vi "Integration Time.vi"(8 "error in (no error)":errorcluster, 10 "Integration Time (0:Short)":u32(ring) items=["Short", "Medium", "Long"], 11 "VISA resource name":refnum<visa-resource-name>) -> (0 "error out":errorcluster, 3 "VISA resource name out":refnum<visa-resource-name>)   [LabVIEW 2017, in "Agilent 4194.lvlib"]
doc: "This function specifies the specifies the integration time."
uses:
  PiezoST/Agilent 4194/Agilent 4194.lvlib
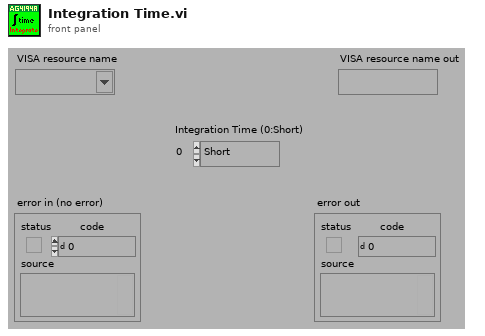
[diagram p1: front panel]
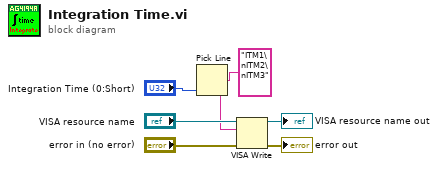
[diagram p0: block diagram]
diagram:
  n1 = Pick Line(multi-line string="ITM1\nITM2\nITM3", line index="Integration Time (0:Short)") -> (output string=w1:string)  [unwired: 1 in]
  n2 = VISA Write(VISA resource name="VISA resource name", write buffer=w1, error in (no error)="error in (no error)") -> (VISA resource name out=→"VISA resource name out":refnum<visa-resource-name>, error out=→"error out":errorcluster)  [unwired: 1 out]
